vi "Adjust Peak Offsets On XY Chart.vi"(8 "error in (no error)":errorcluster, 9 "Echo Range in":dbl caption="Echo Range in (if used)", 10 "AScan+Peaks in":cluster{"timebase":dbl[], "data":u16[]}[](array[cluster])) -> (0 "error out":errorcluster, 2 "AScan+Peaks out":cluster{"timebase":dbl[], "data":u16[]}[](array[cluster]))   [LabVIEW 2026, in "MicroPulse_Driver.lvlib"]
doc: "When Echo Gate is used, it adjusts the time in the peak detection results by removing the offset to the detected first echo. However, when diplayed on a XY chart with the full A-Scan display, the peaks appear in the wrong place. This VI replaces to time offset that was subtracted so that the peaks display in the correct place on the chart."
uses:
  MicroPulse_Driver.lvlib
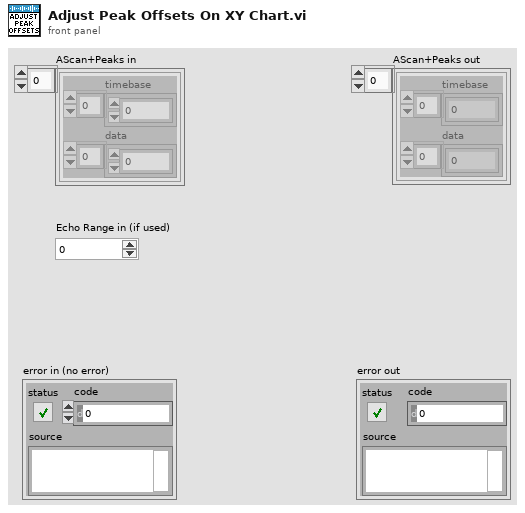
[diagram p1: front panel]
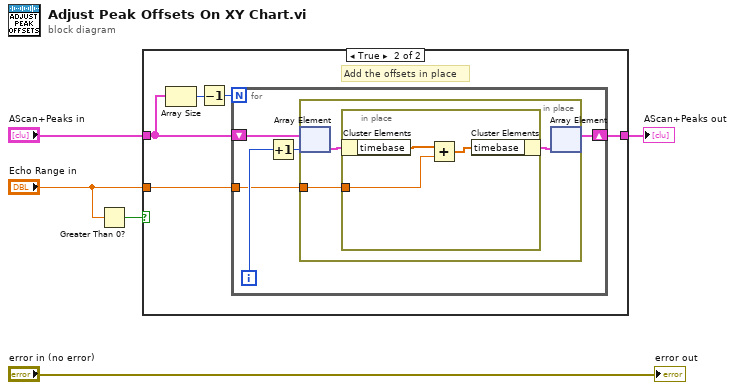
[diagram p0: block diagram]
diagram:
  n1 = Greater Than 0?(x="Echo Range in") -> (x > 0?=w1:bool)
  n2 = case shown="True" w1 {
    tunnel: "AScan+Peaks in" -> [w6 w9]
    tunnel: [w6 w8] -> w4
    tunnel: "Echo Range in" -> [_ w7]
    frame False {
    }
    frame True {
      # "Add the offsets in place"
      n3 = Array Size(array=w9) -> (size(s)=w11:i32)
      n4 = Decrement(x=w11) -> (x-1=w10:i32)
      n5 = for {
        N: w10 -> [_]
        shift-right: [w13] -> w8
        shift-left: w9 -> [w16]
        tunnel: w7 -> [w12]
        i -> [w14]
        n6 = Increment(x=w14) -> (x+1=w15:i32)
        n7 = in-place {
          in-place-border: w12 -> [w18]
          n8 = in-place-array #1(w16, w15) -> (w19:cluster{"timebase":dbl[], "data":u16[]})
          n9 = in-place {
            in-place-border: w18 -> [w21]
            n10 = in-place-cluster #2(w19) -> ("timebase"=w22:dbl[])
            n11 = Add(x=w22, y=w21) -> (x+y=w20:dbl[])
            n12 = in-place-cluster #2("timebase"=w20) -> (w17:cluster{"timebase":dbl[], "data":u16[]})
          }
          n13 = in-place-array #1(w17) -> (w13:cluster{"timebase":dbl[], "data":u16[]}[])  [unwired: 1 out]
        }
      }
    }
  }
  "AScan+Peaks out" <- w4
  "error out" <- "error in (no error)"
